vi "fromXML.vi"(8 "error in (no error)":errorcluster, 9 "xmlPath":string, 10 "channel_configXML":refnum<class "NativeXML.lvclass">, 11 "DigitalChannel in":refnum<class "DigitalChannel.lvclass">) -> (0 "error out":errorcluster, 3 "DigitalChannel out":refnum<class "DigitalChannel.lvclass">)   [LabVIEW 2009, in "Tools.lvlib" / "DatabaseHelpers.lvlib" / "DigitalChannel.lvclass"]
uses:
  DigitalChannel.lvclass
  NativeXML/NativeXML.lvclass
  Channel.lvclass
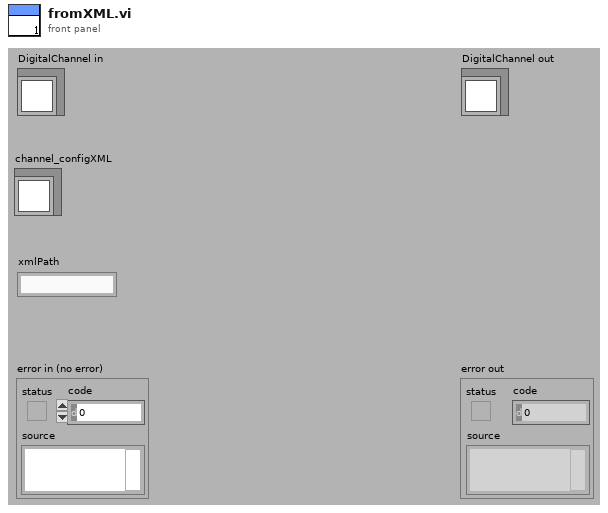
[diagram p1: front panel]
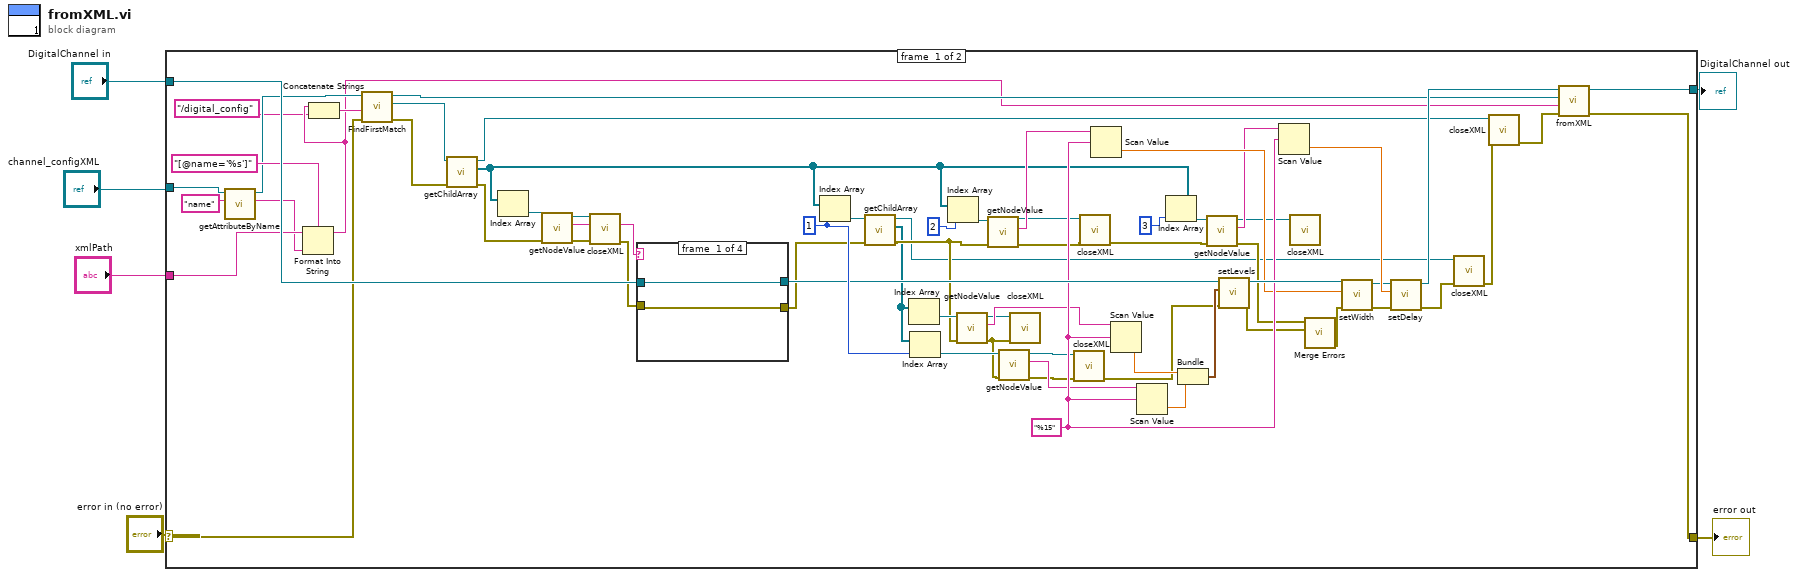
[diagram p0: block diagram]
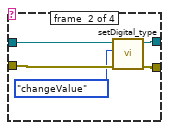
[diagram p2: hidden frame]
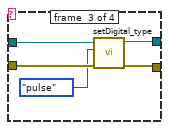
[diagram p3: hidden frame]
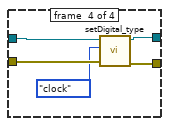
[diagram p4: hidden frame]
diagram:
  n1 = case shown="No Error" "error in (no error)" {
    selector: "error in (no error)" -> [w11 w90]
    tunnel: [w37 w90] -> w6
    tunnel: [w56 w91] -> w5
    tunnel: "channel_configXML" -> [w18 _]
    tunnel: "DigitalChannel in" -> [w57 w91]
    tunnel: "xmlPath" -> [w17 _]
    frame #0 {
      w65 = "%15"
      w72 = 1
      n2 = call "getAttributeByName.vi"("name"="name", "NativeXML in"=w18) -> ("Attribute String"=w16:string, "NativeXML out"=w14:refnum<class "NativeXML.lvclass">)  [unwired: 7 in, 1 out]
      n3 = Format Into String(format string="[@name='%s']", initial string=w17, w16) -> (resulting string=w8:string)  [unwired: 1 in, 1 out]
      n4 = Concatenate Strings(w8, "/digital_config") -> (w9:string)
      n5 = call "FindFirstMatch.vi"("error in (no error)"=w11, "xPath"=w9, "NativeXML in"=w14) -> ("error out"=w10:errorcluster, "NativeXML match"=w12:refnum<class "NativeXML.lvclass">, "NativeXML out"=w13:refnum<class "NativeXML.lvclass">)  [unwired: 6 in]
      n6 = call "getChildArray.vi"("error in (no error)"=w10, "NativeXML in"=w12) -> ("error out"=w52:errorcluster, "childArray"=w38:refnum<class "NativeXML.lvclass">[], "NativeXML out"=w20:refnum<class "NativeXML.lvclass">)  [unwired: 7 in]
      n7 = Index Array(array=w38) -> (element=w54:refnum<class "NativeXML.lvclass">)  [unwired: 1 in]
      n8 = call "getNodeValue.vi"("error in (no error)"=w52, "NativeXML in"=w54) -> ("error out"=w35:errorcluster, "Value"=w53:string, "NativeXML out"=w36:refnum<class "NativeXML.lvclass">)  [unwired: 7 in]
      n9 = call "closeXML.vi"("error in (no error)"=w35, "NativeXML in"=w36) -> ("error out"=w34:errorcluster)  [unwired: 9 in]
      n10 = case shown="\"changeValue\"" w53 {
        tunnel: w57 -> [w74 w79 w84 w89]
        tunnel: w34 -> [w73 w78 w83 w88]
        tunnel: [w74 w76 w81 w86] -> w69
        tunnel: [w73 w75 w80 w85] -> w51
        frame #0 {
        }
        frame #1 {
          n11 = call "setDigital_type.vi"("error in (no error)"=w78, "digital_type"=enum16{"changeValue", "pulse", "clock"}."changeValue", "DigitalChannel.lvclass in"=w79) -> ("error out"=w75:errorcluster, "DigitalChannel.lvclass out"=w76:refnum<class "DigitalChannel.lvclass">)  [unwired: 7 in]
        }
        frame #2 {
          n12 = call "setDigital_type.vi"("error in (no error)"=w83, "digital_type"=enum16{"changeValue", "pulse", "clock"}."pulse", "DigitalChannel.lvclass in"=w84) -> ("error out"=w80:errorcluster, "DigitalChannel.lvclass out"=w81:refnum<class "DigitalChannel.lvclass">)  [unwired: 7 in]
        }
        frame #3 {
          n13 = call "setDigital_type.vi"("error in (no error)"=w88, "digital_type"=enum16{"changeValue", "pulse", "clock"}."clock", "DigitalChannel.lvclass in"=w89) -> ("error out"=w85:errorcluster, "DigitalChannel.lvclass out"=w86:refnum<class "DigitalChannel.lvclass">)  [unwired: 7 in]
        }
      }
      n14 = Index Array(array=w38, index=w72) -> (element=w50:refnum<class "NativeXML.lvclass">)
      n15 = call "getChildArray.vi"("error in (no error)"=w51, "NativeXML in"=w50) -> ("error out"=w43:errorcluster, "childArray"=w39:refnum<class "NativeXML.lvclass">[], "NativeXML out"=w24:refnum<class "NativeXML.lvclass">)  [unwired: 7 in]
      n16 = Index Array(array=w39) -> (element=w49:refnum<class "NativeXML.lvclass">)  [unwired: 1 in]
      n17 = Index Array(array=w39, index=w72) -> (element=w47:refnum<class "NativeXML.lvclass">)
      n18 = Index Array(array=w38, index=2) -> (element=w42:refnum<class "NativeXML.lvclass">)
      n19 = call "getNodeValue.vi"("error in (no error)"=w43, "NativeXML in"=w49) -> ("error out"=w32:errorcluster, "Value"=w48:string, "NativeXML out"=w33:refnum<class "NativeXML.lvclass">)  [unwired: 7 in]
      n20 = call "getNodeValue.vi"("error in (no error)"=w43, "NativeXML in"=w42) -> ("error out"=w28:errorcluster, "Value"=w41:string, "NativeXML out"=w27:refnum<class "NativeXML.lvclass">)  [unwired: 7 in]
      n21 = call "getNodeValue.vi"("error in (no error)"=w32, "NativeXML in"=w47) -> ("error out"=w30:errorcluster, "Value"=w46:string, "NativeXML out"=w31:refnum<class "NativeXML.lvclass">)  [unwired: 7 in]
      n22 = call "closeXML.vi"("error in (no error)"=w32, "NativeXML in"=w33) -> ()  [unwired: 9 in, 1 out]
      n23 = call "closeXML.vi"("error in (no error)"=w30, "NativeXML in"=w31) -> ("error out"=w29:errorcluster)  [unwired: 9 in]
      n24 = call "closeXML.vi"("error in (no error)"=w28, "NativeXML in"=w27) -> ("error out"=w26:errorcluster)  [unwired: 9 in]
      n25 = Scan Value(string=w41, format string=w65) -> (value=w63:dbl)  [unwired: 1 in, 1 out]
      n26 = Scan Value(string=w48, format string=w65) -> (value=w71:dbl)  [unwired: 1 in, 1 out]
      n27 = Scan Value(string=w46, format string=w65) -> (value=w70:dbl)  [unwired: 1 in, 1 out]
      n28 = Index Array(array=w38, index=3) -> (element=w45:refnum<class "NativeXML.lvclass">)
      n29 = Bundle(w71, w70) -> (w68:cluster{dbl, dbl})  [unwired: 1 in]
      n30 = call "getNodeValue.vi"("error in (no error)"=w26, "NativeXML in"=w45) -> ("error out"=w40:errorcluster, "Value"=w44:string, "NativeXML out"=w25:refnum<class "NativeXML.lvclass">)  [unwired: 7 in]
      n31 = call "setLevels.vi"("error in (no error)"=w29, "levels"=w68, "DigitalChannel.lvclass in"=w69) -> ("error out"=w61:errorcluster, "DigitalChannel.lvclass out"=w67:refnum<class "DigitalChannel.lvclass">)  [unwired: 7 in]
      n32 = Scan Value(string=w44, format string=w65) -> (value=w64:dbl)  [unwired: 1 in, 1 out]
      n33 = call "closeXML.vi"("NativeXML in"=w25) -> ()  [unwired: 10 in, 1 out]
      n34 = call <vilib>:"Merge Errors.vi"("error in 2 (no error)"=w61, "error in 1 (no error)"=w40) -> ("error out"=w60:errorcluster)  [unwired: 5 in]
      n35 = call "setWidth.vi"("error in (no error)"=w60, "width"=w63, "DigitalChannel.lvclass in"=w67) -> ("error out"=w62:errorcluster, "DigitalChannel.lvclass out"=w59:refnum<class "DigitalChannel.lvclass">)  [unwired: 7 in]
      n36 = call "setDelay.vi"("error in (no error)"=w62, "delay"=w64, "DigitalChannel.lvclass in"=w59) -> ("error out"=w23:errorcluster, "DigitalChannel.lvclass out"=w55:refnum<class "DigitalChannel.lvclass">)  [unwired: 7 in]
      n37 = call "closeXML.vi"("error in (no error)"=w23, "NativeXML in"=w24) -> ("error out"=w22:errorcluster)  [unwired: 9 in]
      n38 = call "closeXML.vi"("error in (no error)"=w22, "NativeXML in"=w20) -> ("error out"=w21:errorcluster)  [unwired: 9 in]
      n39 = call-parent "fromXML.vi"("error in (no error)"=w21, "xmlPath"=w8, "channel_configXML"=w13, "Channel in"=w55) -> ("error out"=w37:errorcluster, "Channel out"=w56:refnum<class "DigitalChannel.lvclass">)  [unwired: 6 in]
    }
    frame #1 {
    }
  }
  "error out" <- w6
  "DigitalChannel out" <- w5
